vi "CONVERSOR.vi"(2 "String":string) -> (6 "inteiro":i32, 7 "float":dbl, 9 "String":string, 10 "boolean":bool)   [LabVIEW 2019]
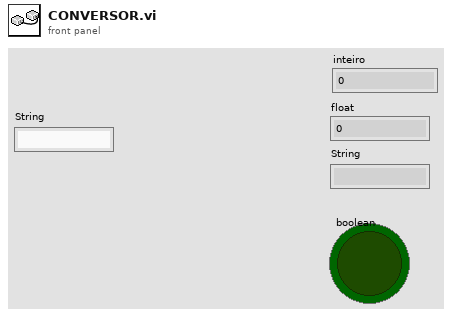
[diagram p1: front panel]
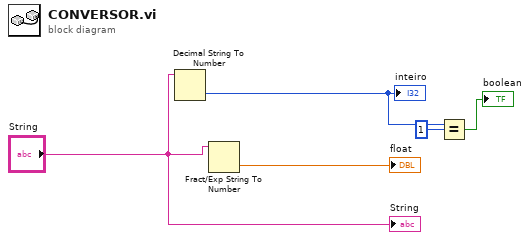
[diagram p0: block diagram]
diagram:
  n1 = Decimal String To Number(string="String") -> (number=w3:i32)  [unwired: 2 in, 1 out]
  "inteiro" <- w3
  n2 = Fract/Exp String To Number(string="String") -> (number=→"float":dbl)  [unwired: 3 in, 1 out]
  n3 = Equal?(x=w3, y=1) -> (x = y?=→"boolean":bool)
  "String" <- "String"
